vi "WF phase diversity_MATLAB_Correction_loop_AndorSDK.vi"() -> ()   [LabVIEW 2018]
uses:
  <userlib>/WaveKit.lib/Controls/Wavefront Corrector states - ONE.ctl
  <userlib>/WaveKit.lib/Classes/WavefrontCorrector/WavefrontCorrector.lvclass
  <userlib>/WaveKit.lib/Classes/WavefrontCorrectorSet/WavefrontCorrectorSet.lvclass
  <vilib>/Analysis/1siggen.llb/Ramp Pattern by Samples.vi
  <vilib>/Utility/file.llb/Read From Spreadsheet File (DBL).vi
  <vilib>/Analysis/1siggen.llb/Ramp Pattern by Delta.vi
  <vilib>/Analysis/NI_AALBase.lvlib
panel:
  out "Error out tbd":errorcluster
  in  "Tab Control":T1(tab)
  in  "Offset command file":path=path "D:/SystemAlignment/system_aberration_20200627.dat"
  in  "Initial haso file":path=path "D:/SystemAlignment/system_aberration_residual_20200627.has"
  out "# of Phase":i32
  in  "DM configuration file":path=path "C:/Program Files (x86)/Imagine Optic/Configuration Files/WaveFrontCorrector_mirao52-e_0326.dat"
  out "DM Initial State":T2[](array[typedef])
  out "DM ActuatorsNumber":i32
  out "Error out":errorcluster
  in  "Error in":errorcluster
  in  "EMCCD trigger port":tag="Dev1/port0/line0"
  in  "Cooler set to Temperature":i32=-60
  in  "Trigger":u32(ring)=1 items=["Internal", "External"]
  out "Return from CheckTimings":u32
  out "Calculated Exposure Value":sgl format="%.2f"
  out "Return from SetTemperature":u32
  out "Cooling":i32
  out "Return from Initialize":u32
  out "Detector X Pixels":i32
  out "Detector Y Pixels":i32
  in  "Initialize EMCCD?":bool=TRUE
  in  "Turn off cooler when finished?":bool
  in  "Initial Zer coeff":dbl[](array[numeric])=[0.2, 0.2]
  in  "Initial Zer index":dbl[](array[numeric])=[4.0, 5.0]
  out "Initial Zer coeff\nRandomly generated":dbl[](array[numeric])
  out "Initial Zer index (starting from 4)\nrandomly generated":dbl[](array[numeric])
  in  "aberration tolerance":dbl=0.1 format="%#_13g"
  in  "aberration threshold":dbl=0.25 format="%#_13g"
  in  "?":enum16{"input manually ", "randomly generated"}(ring)
  in  "max random order":i64=9
  in  "NOT YET: Data Acquisition Iteration #":i32=1
  in  "Zern index in 2":i32[](array[numeric])=[3, 4, 5, 6, 7, 8]
  in  "Zern coef in 2":sgl[](array[numeric])=[0.2, 0.5, 0.0, 0.0, 0.0, 0.0]
  in  "Zern index in 3":i32[](array[numeric])=[3, 4, 5, 6, 7, 8]
  in  "Zern coef in 3":sgl[](array[numeric])=[0.2, 0.0, 0.0, 0.0, 0.0, 0.0]
  in  "Zern index in 4":i32[](array[numeric])=[3, 4, 5, 6, 7, 8]
  in  "Zern coef in 4":sgl[](array[numeric])=[0.2, 0.0, 0.0, 0.0, 0.0, 0.0]
  in  "Zern index in 5":i32[](array[numeric])=[3, 4, 5, 6, 7, 8]
  in  "Zern coef in 5":sgl[](array[numeric])=[0.0, 0.0, 0.0, 0.0, 0.0, -0.2]
  in  "Andor Picture/notes save to path":path=path "D:/YD/test/test1"
  in  "base name (no \"_\" in the end)":string="beads_test"
  in  "Pics/phase":dbl=2.0
  in  "camera exposure time (s)":string="0.02"
  in  "# of Phase":i32=5
  in  "COMMAND matrix path":path=path "D:/SystemAlignment/CM_20200711_0p5x6.aomc"
  in  "488 shutter":refnum<k7>(container)
  in  "?":bool
  out "phase diversity file name":string
  out "Corrected Picture name":string
  in  "Use GPU":bool=TRUE
  in  "Show Recon":bool=TRUE
  in  "Show Input":bool
  in  "Background Value":u32=310
  in  "Crop Size of image":u32=512
  in  "Gamma Value":dbl=1e-06
  in  "Iteration Number":u32=10
  in  "Zernike Order":u32=21
  in  "Number for average":u32=2
  in  "Number of Phase":u32=2
  in  "Run MATLAB or correction?":bool=TRUE
  in  "Keep Reconstructed Defocus component?":bool
  # "matlab module :\nC:\\Control Software\\LabviewControl\\sub_vis_Wavekit\\recon_zern_fileIO_MATLAB_v2.vi"
  # "Cooler is off for testing"
  # "If Pics/phase is 2:\npicture order:\n\noffset+aberr *2\nphase diversity *8\n\nground truth *1\noffset+aberr *1\ncorrected *2 but the last one cannot be seen in imagej"
  # "Randomly Generate Initial Zernike, enter here:"
  # "Manually input, enter here:"
  # "Andor Camera Settings"
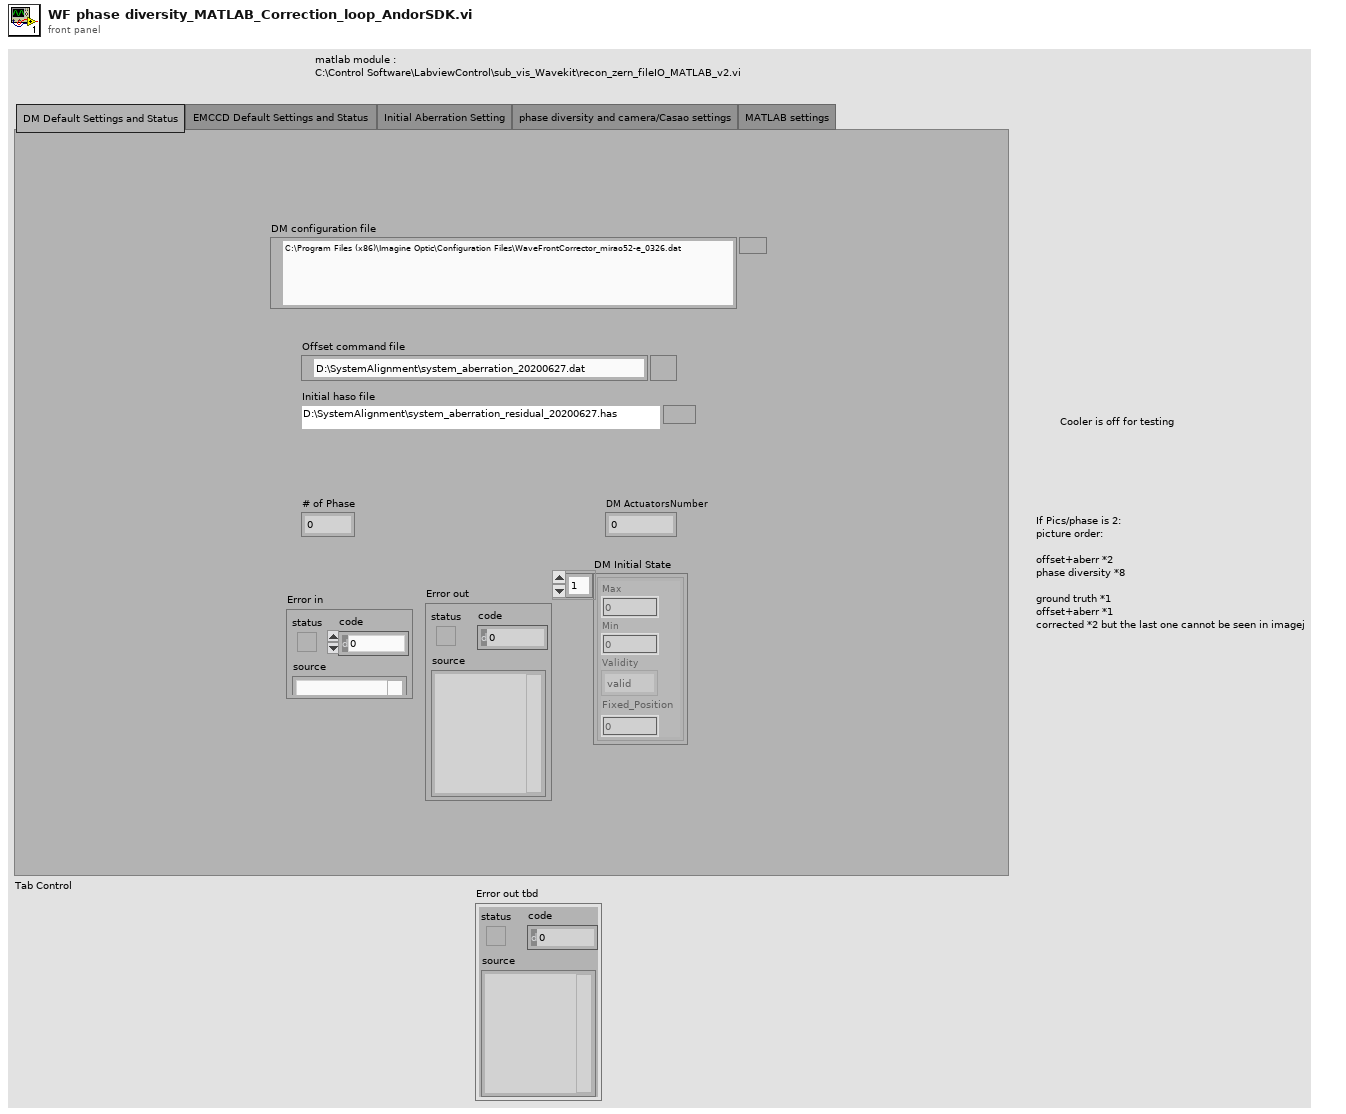
[diagram p1: front panel]
types:
  T1 = enum32{"DM Default Settings and Status", "EMCCD Default Settings and Status ", "Initial Aberration Setting", "phase diversity and camera/Casao settings", "MATLAB settings"}
  T2 = typedef "Wavefront Corrector states - ONE.ctl" = cluster{"Max":sgl, "Min":sgl, "Validity":enum16{"valid", "fixed", "invalid"}, "Fixed_Position":sgl}
  T3 = typedef "Error Code Enum typedef.ctl" = enum32{"N/A (0)", "DRV_ERROR_CODES", "DRV_SUCCESS", "DRV_VXDNOTINSTALLED", "DRV_ERROR_SCAN", "DRV_ERROR_CHECK_SUM", "DRV_ERROR_FILELOAD", "DRV_UNKNOWN_FUNC", "DRV_ERROR_VXD_INIT", "DRV_ERROR_ADDRESS", "DRV_ERROR_PAGELOCK", "DRV_ERROR_PAGEUNLOCK", "DRV_ERROR_BOARDTEST", "DRV_ERROR_ACK", "DRV_ERROR_UP_FIFO", "DRV_ERROR_PATTERN", "N/A (16)", "DRV_ACQUISITION_ERRORS", "DRV_ACQ_BUFFER", "DRV_ACQ_DOWNFIFO_FULL", "DRV_PROC_UNKONWN_INSTRUCTION", "DRV_ILLEGAL_OP_CODE", "DRV_KINETIC_TIME_NOT_MET", "DRV_ACCUM_TIME_NOT_MET", "DRV_NO_NEW_DATA", "N/A (25)", "DRV_SPOOLERROR", "N/A (27)", "N/A (28)", "N/A (29)", "N/A (30)", "N/A (31)", "N/A (32)", "DRV_TEMPERATURE_CODES", "DRV_TEMPERATURE_OFF", "DRV_TEMPERATURE_NOT_STABILIZED", "DRV_TEMPERATURE_STABILIZED", "DRV_TEMPERATURE_NOT_REACHED", "DRV_TEMPERATURE_OUT_RANGE", "DRV_TEMPERATURE_NOT_SUPPORTED", "DRV_TEMPERATURE_DRIFT", "N/A (41)", "N/A (42)", "N/A (43)", "N/A (44)", "N/A (45)", "N/A (46)", "N/A (47)", "N/A (48)", "DRV_GENERAL_ERRORS", "DRV_INVALID_AUX", "DRV_COF_NOTLOADED", "DRV_FPGAPROG", "DRV_FLEXERROR", "DRV_GPIBERROR", "N/A (55)", "N/A (56)", "N/A (57)", "N/A (58)", "N/A (59)", "N/A (60)", "N/A (61)", "N/A (62)", "N/A (63)", "DRV_DATATYPE", "DRV_DRIVER_ERRORS", "DRV_P1INVALID", "DRV_P2INVALID", "DRV_P3INVALID", "DRV_P4INVALID", "DRV_INIERROR", "DRV_COFERROR", "DRV_ACQUIRING", "DRV_IDLE", "DRV_TEMPCYCLE", "DRV_NOT_INITIALIZED", "DRV_P5INVALID", "DRV_P6INVALID", "DRV_INVALID_MODE", "DRV_INVALID_FILTER", "DRV_I2CERRORS", "DRV_I2CDEVNOTFOUND", "DRV_I2CTIMEOUT", "DRV_P7INVALID", "N/A (84)", "N/A (85)", "N/A (86)", "N/A (87)", "N/A (88)", "N/A (89)", "DRV_IOCERROR", "DRV_VRMVERSIONERROR"}
  T4 = typedef "NI_Matrix.lvlib/RealMatrix.ctl" = dbl[][]
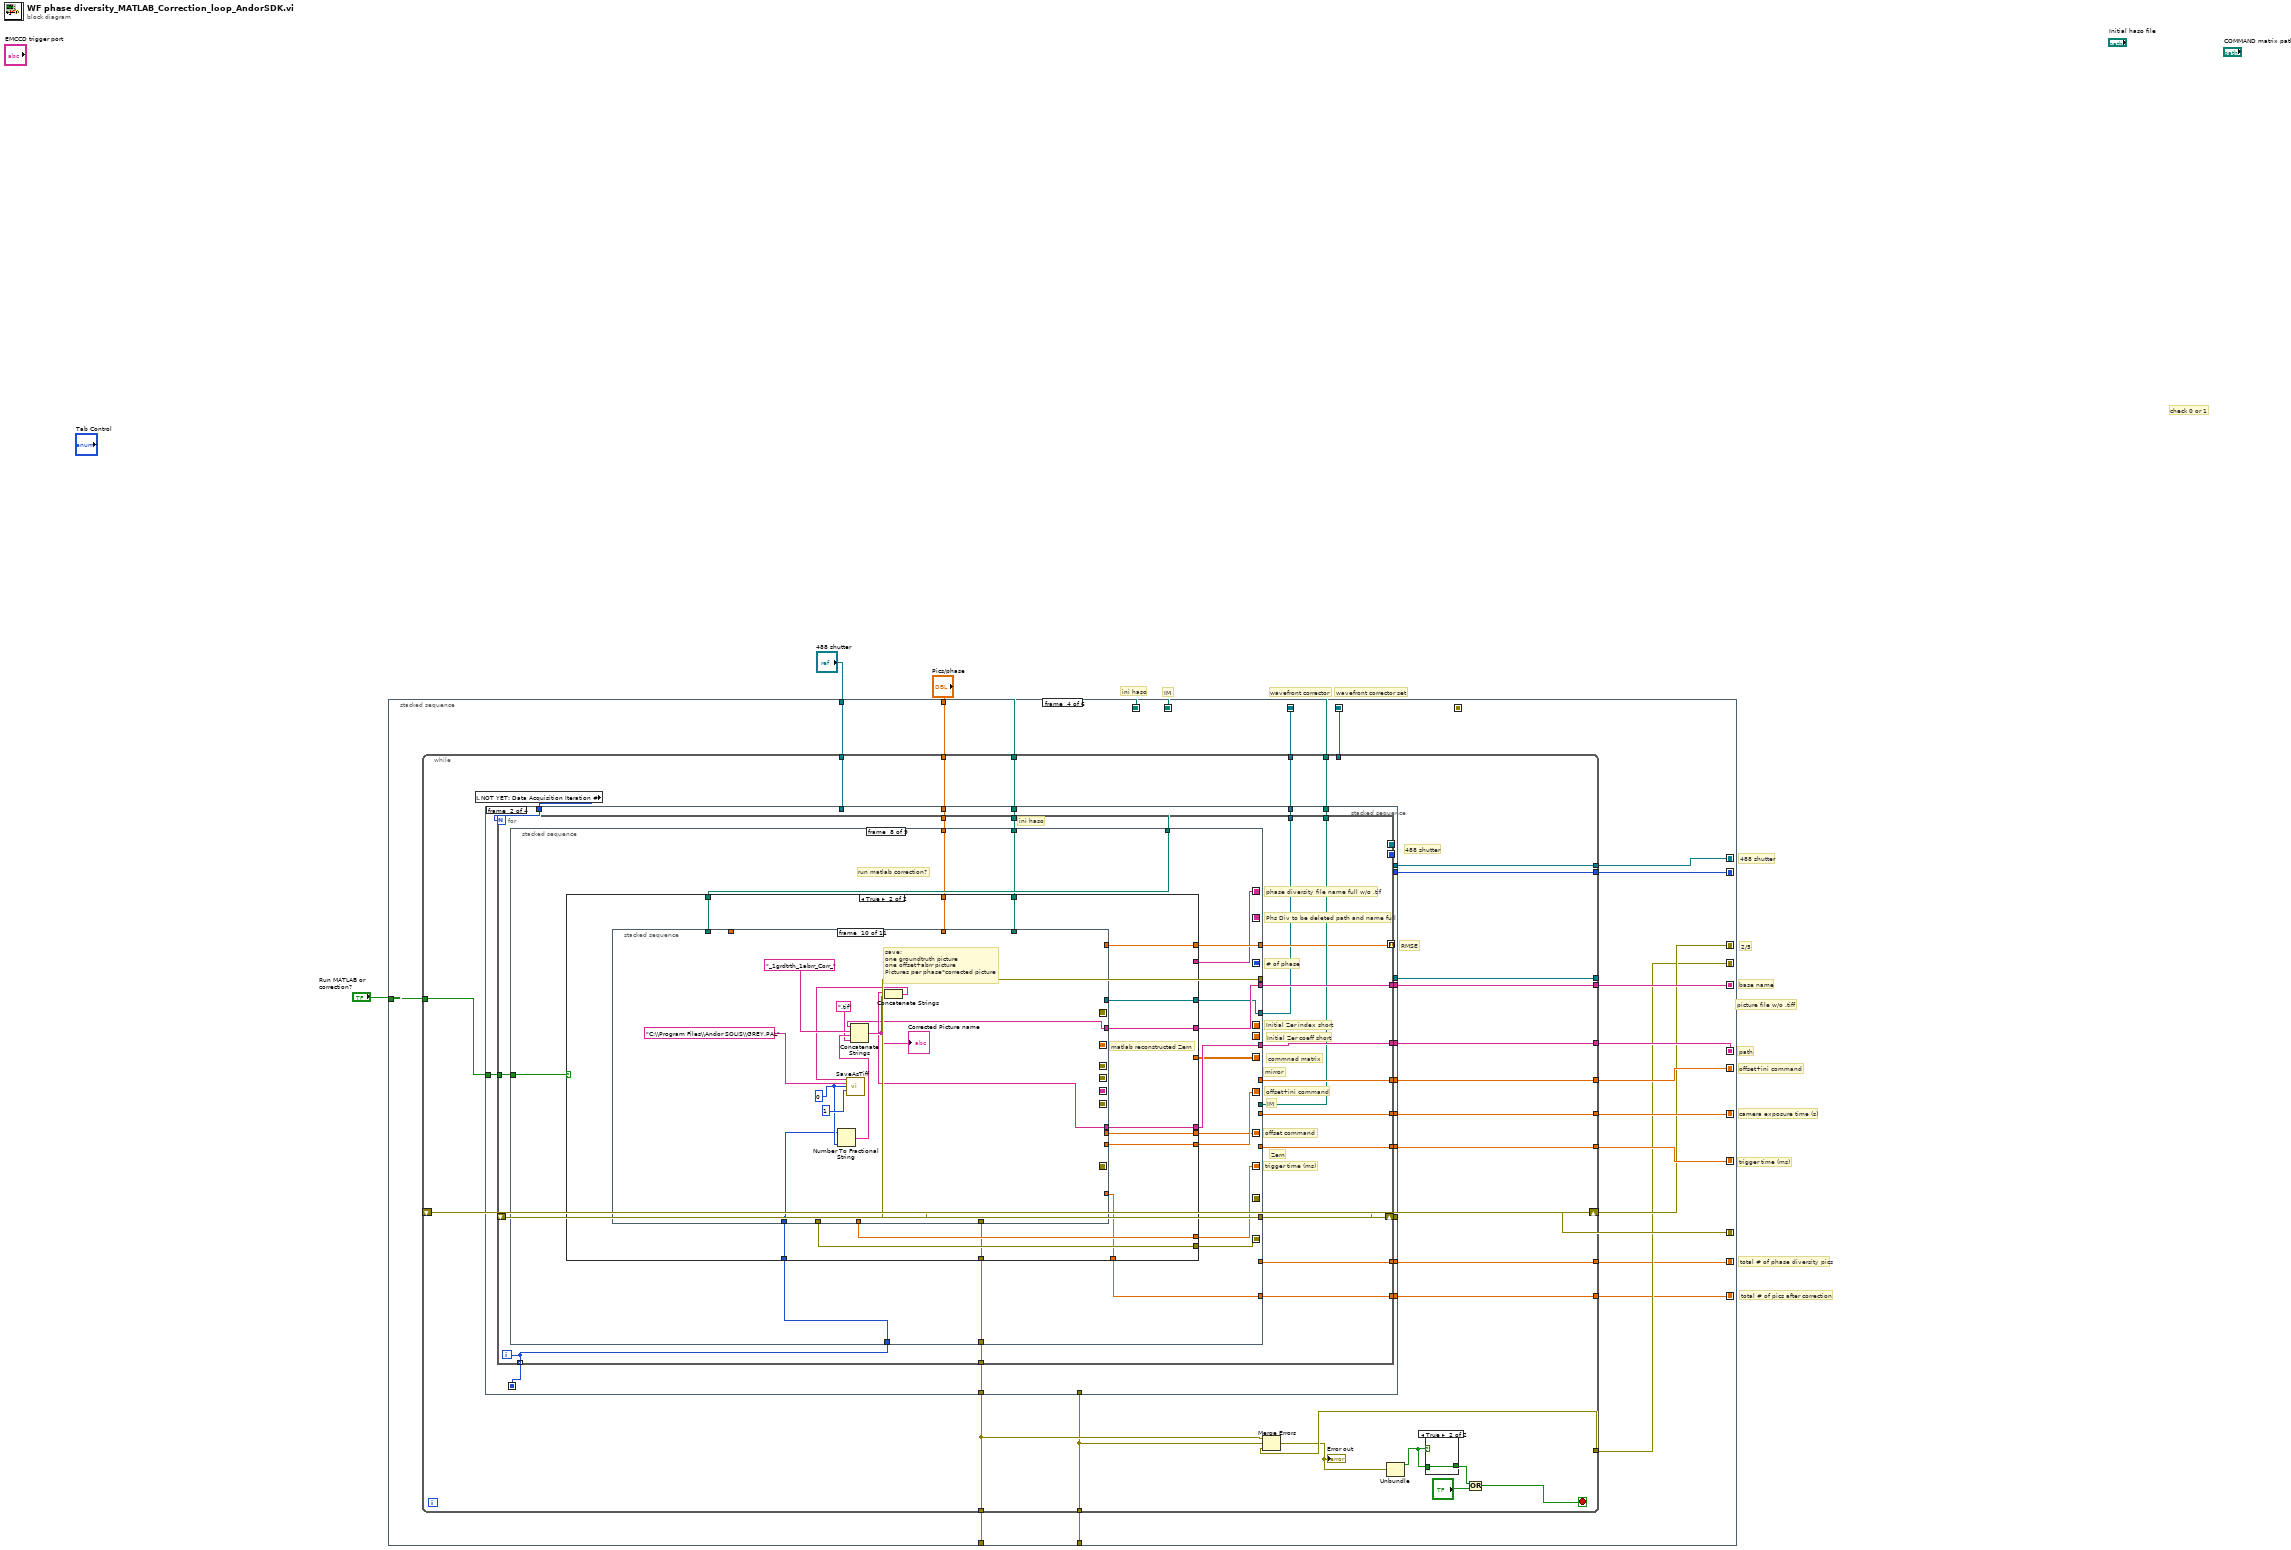
[diagram p0: block diagram]
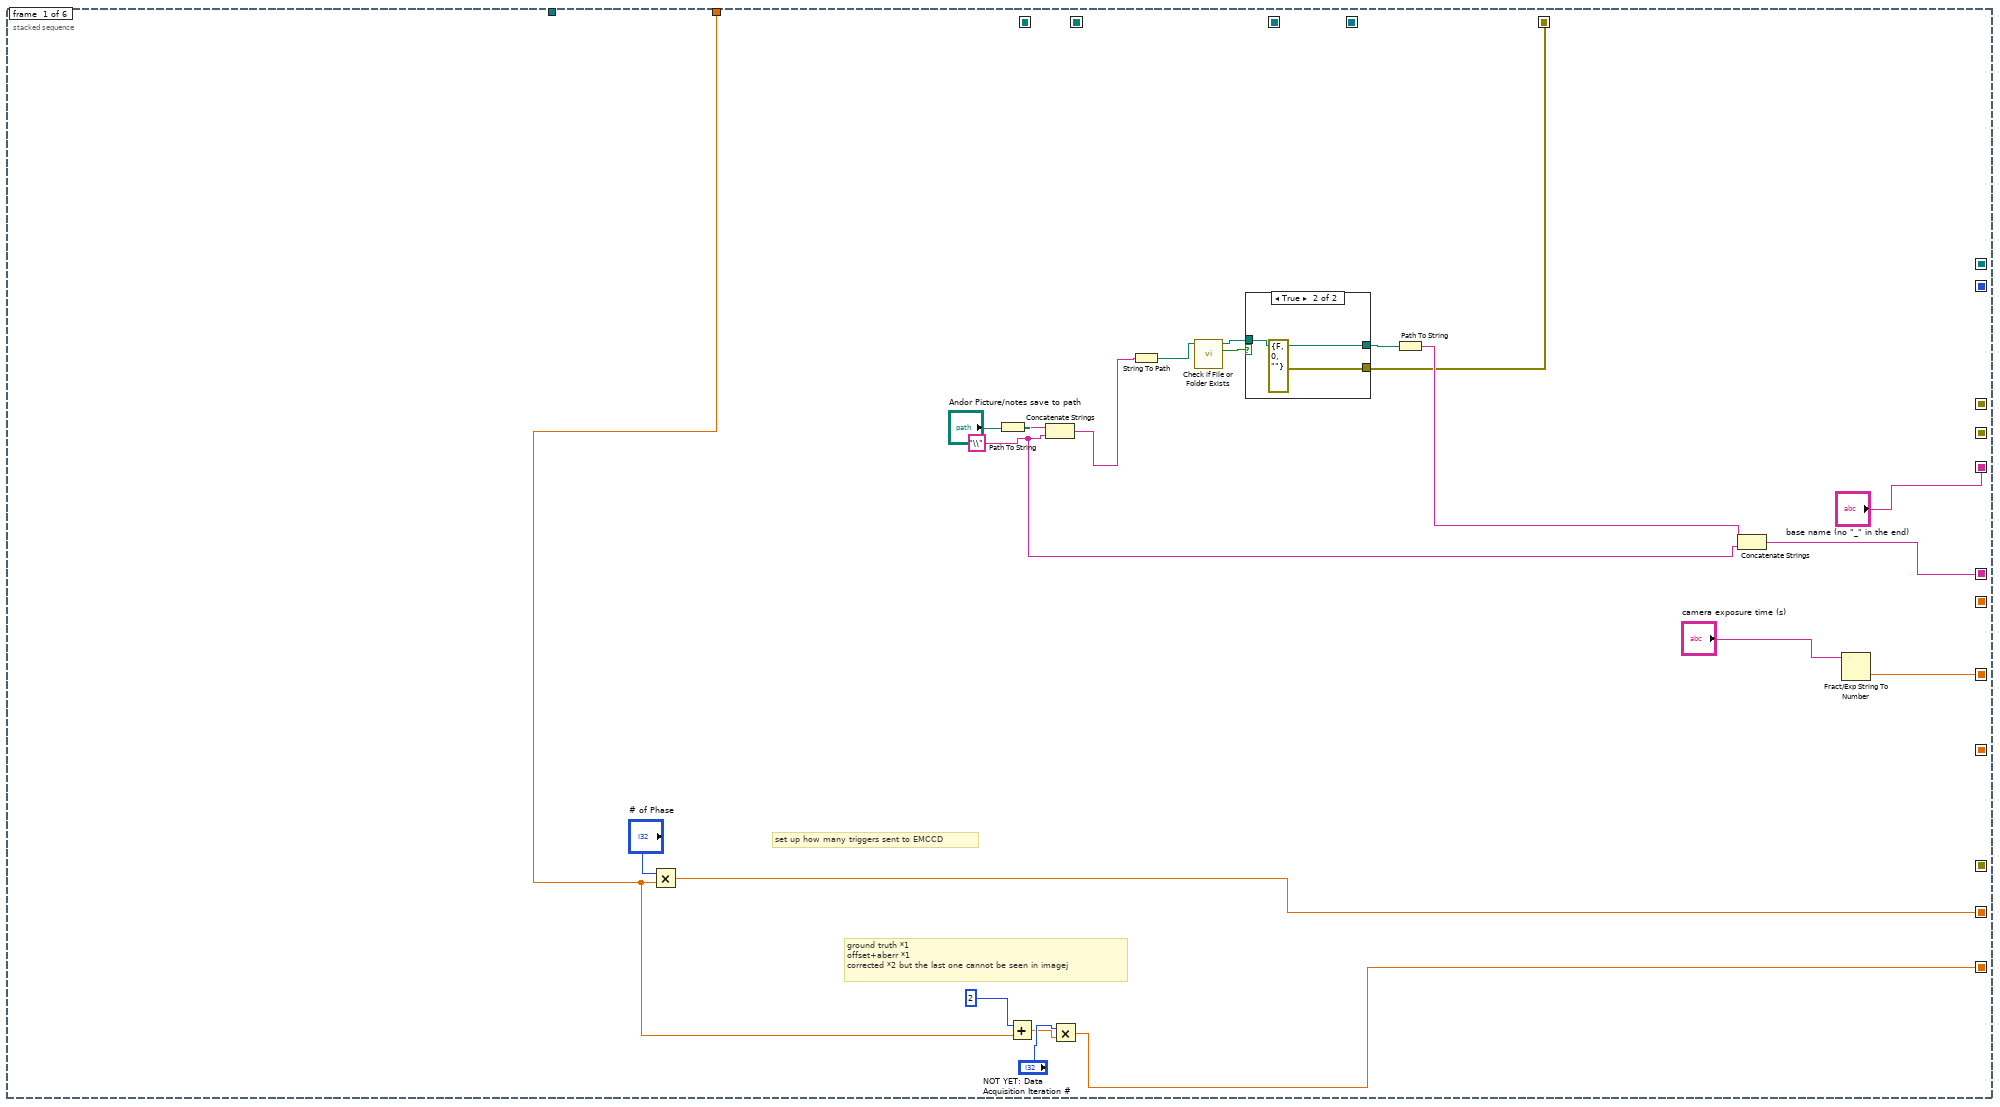
[diagram p2: hidden frame]
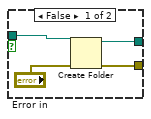
[diagram p3: hidden frame]
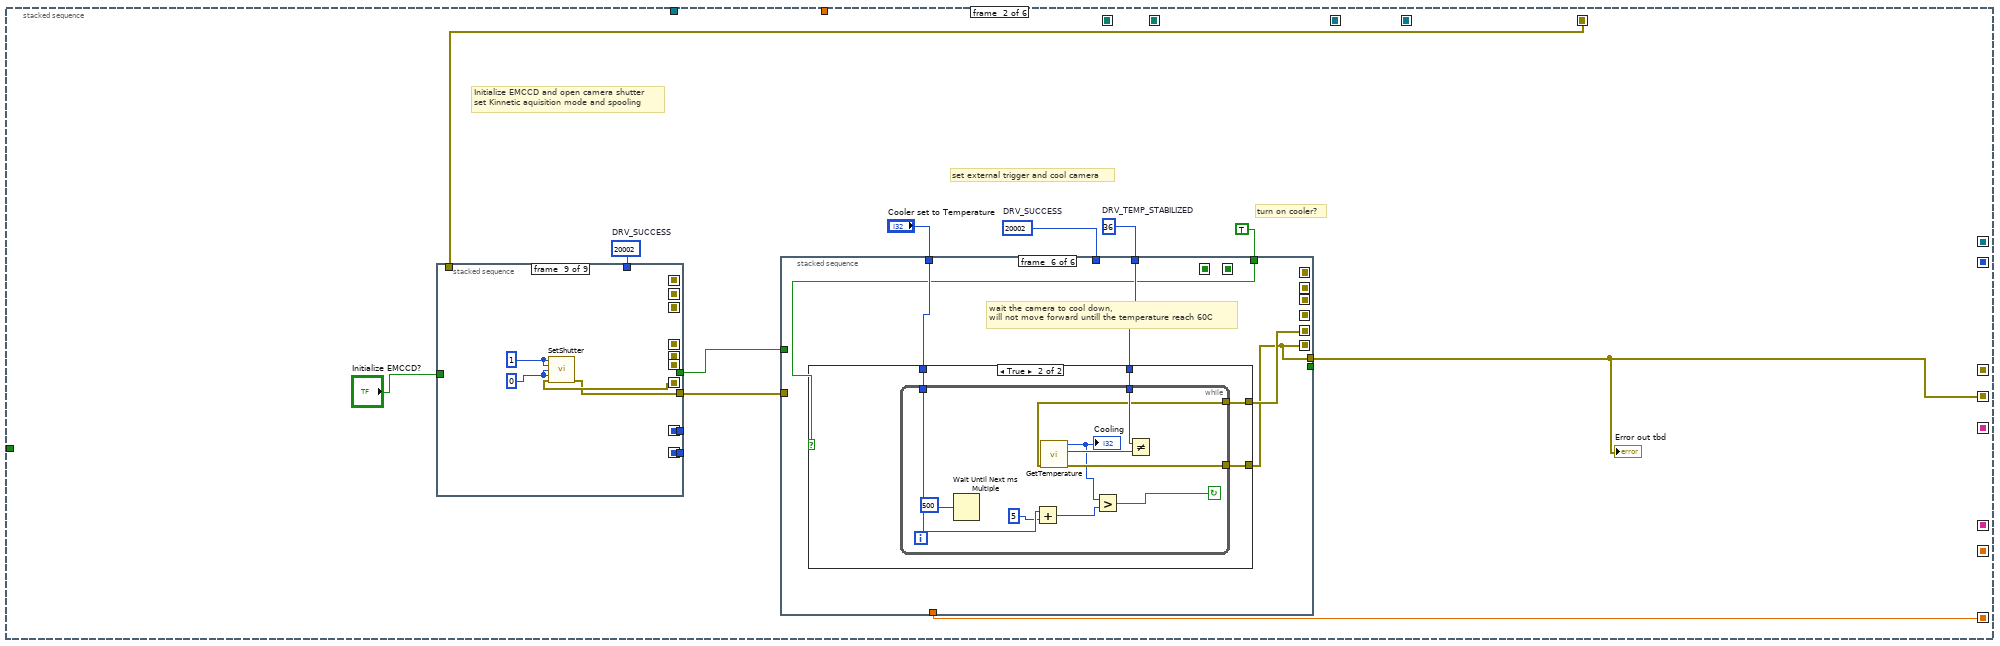
[diagram p4: hidden frame]
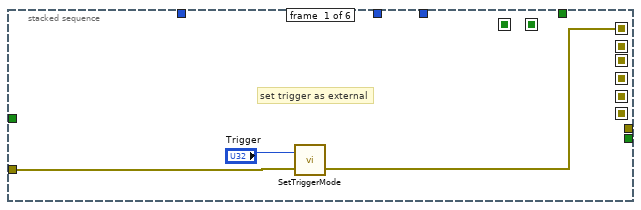
[diagram p5: hidden frame]
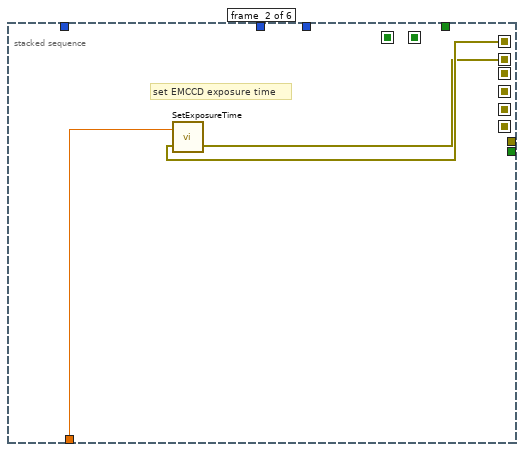
[diagram p6: hidden frame]
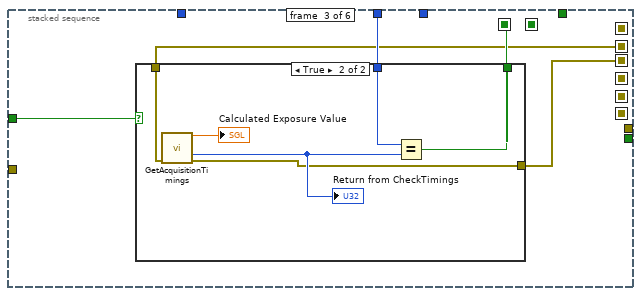
[diagram p7: hidden frame]
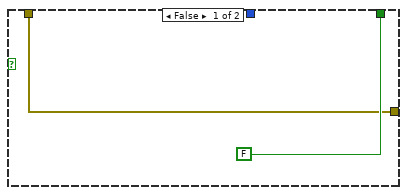
[diagram p8: hidden frame]
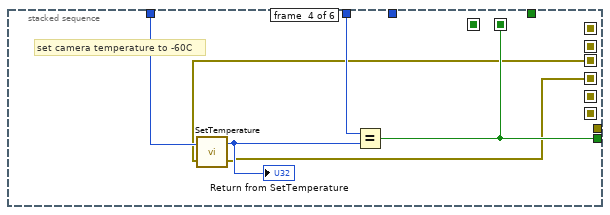
[diagram p9: hidden frame]
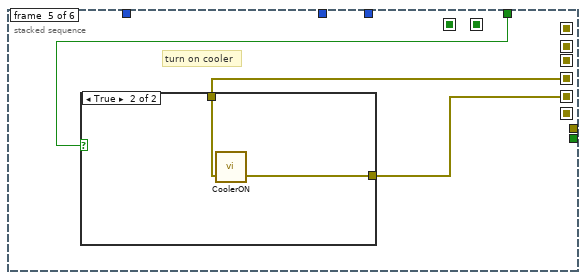
[diagram p10: hidden frame]
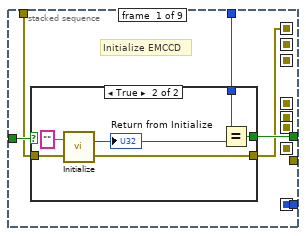
[diagram p13: hidden frame]
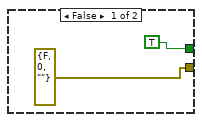
[diagram p14: hidden frame]
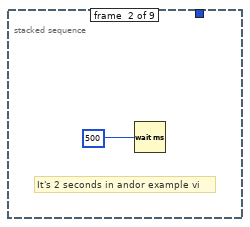
[diagram p15: hidden frame]
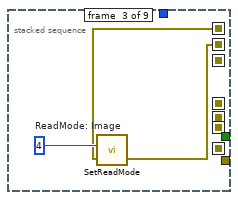
[diagram p16: hidden frame]
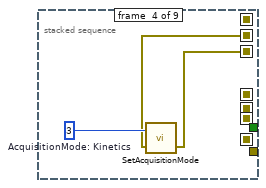
[diagram p17: hidden frame]
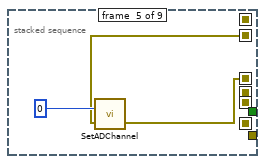
[diagram p18: hidden frame]
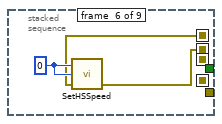
[diagram p19: hidden frame]
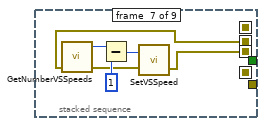
[diagram p20: hidden frame]
diagram:
  # "2/5"
  # "total # of phase diversity pics"
  # "picture file w/o .tiff"
  # "total # of pics after correction"
  # "wavefront corrector set"
  # "wavefront corrector"
  # "488 shutter"
  # "trigger time (ms)"
  # "offset+ini command"
  # "camera exposure time (s)"
  # "IM"
  # "ini haso"
  # "path"
  # "base name"
  # "check 0 or 1"
  n1 = stacked-sequence {
    seq-local: [w5 _ _ _ _ _] -> [_ _ _ w174 _ _]
    seq-local: ["base name (no \"_\" in the end)" _ _ _ _ _] -> [_ _ _ w173 _ _]
    seq-local: [_ _ w154 _ _ _] -> [_ _ _ w172 _ _]
    seq-local: [_ _ w153 _ _ _] -> [_ _ _ w167 _ _]
    seq-local: [w19 _ _ _ _ _] -> [_ w35 _ w171 _ _]
    seq-local: [_ _ w139 _ _ _] -> [_ _ _ w159 _ _]
    seq-local: [_ _ _ w170 _ _] -> [_ _ _ _ _ _]
    seq-local: [_ _ _ w169 _ _] -> [_ _ _ _ _ _]
    seq-local: [_ _ _ w168 _ _] -> [_ _ _ _ _ w643]
    seq-local: [_ _ _ w162 _ _] -> [_ _ _ _ _ _]
    seq-local: [_ _ _ w165 _ _] -> [_ _ _ _ _ _]
    seq-local: [_ _ w138 _ _ _] -> [_ _ _ w160 _ w645]
    seq-local: [_ _ w137 _ _ _] -> [_ _ _ w158 _ w644]
    seq-local: [w16 _ _ _ _ _] -> [_ _ _ w155 _ _]
    seq-local: [_ w31 _ _ _ _] -> [_ _ w136 w157 _ _]
    seq-local: [w15 _ _ _ _ _] -> [_ _ _ w156 _ _]
    seq-local: [w4 _ _ _ _ _] -> [_ w32 _ _ _ _]
    tunnel: "Pics/phase" -> [w13 _ _ w175 _ _]
    tunnel: "Run MATLAB or correction?" -> [_ _ _ w166 _ _]
    tunnel: [_ _ _ w164 _ _] -> _
    tunnel: [_ _ _ w163 _ _] -> _
    tunnel: "488 shutter" -> [_ _ _ w161 _ w646]
    frame #0 {
      w6 = "\\"
      # "set up how many triggers sent to EMCCD"
      # "ground truth *1\noffset+aberr *1\ncorrected *2 but the last one cannot be seen in imagej"
      n2 = Multiply(x="# of Phase", y=w13) -> (x*y=w15:dbl)
      n3 = Path To String(path="Andor Picture/notes save to path") -> (string=w21:string)
      n4 = Add(x=2, y=w13) -> (x+y=w17:dbl)
      n5 = Concatenate Strings(w21, w6) -> (w8:string)
      n6 = Multiply(x="NOT YET: Data Acquisition Iteration #", y=w17) -> (x*y=w16:dbl)
      n7 = String To Path(string=w8) -> (path=w12:path)
      n8 = call <vilib>:"Check if File or Folder Exists.vi"("path"=w12) -> ("file or folder exists?"=w10:bool, "dup path"=w11:path)  [unwired: 8 in, 1 out]
      n9 = case shown="True" w10 {
        tunnel: w11 -> [w28 w30]
        tunnel: [w27 w30] -> w9
        tunnel: [w25 errorcluster {"status"=FALSE, "code"=0, "source"=""} ("Error in 3")] -> w4
        frame False {
          n10 = Create Folder(path (use dialog)=w28, error in="Error in") -> (created path=w27:path, error out=w25:errorcluster)  [unwired: 1 in, 1 out]
        }
        frame True {
        }
      }
      n11 = Path To String(path=w9) -> (string=w7:string)
      n12 = Concatenate Strings(w7, w6) -> (w5:string)
      n13 = Fract/Exp String To Number(string="camera exposure time (s)") -> (number=w19:dbl)  [unwired: 3 in, 1 out]
    }
    frame #1 {
      w37 = 36  # DRV_TEMP_STABILIZED
      w39 = 20002  # DRV_SUCCESS
      w41 = 20002  # DRV_SUCCESS
      # "turn on cooler?"
      # "set external trigger and cool camera"
      # "Initialize EMCCD and open camera shutter\nset Kinnetic aquisition mode and spooling"
      n14 = stacked-sequence {
        seq-local: [_ _ _ _ _ _ _ w125 _] -> [_ _ _ _ _ _ _ _ _]
        seq-local: [_ _ _ _ _ _ _ w127 _] -> [_ _ _ _ _ _ _ _ _]
        seq-local: [w95 _ _ _ _ _ _ _ _] -> [_ _ w108 _ _ _ _ _ _]
        seq-local: [_ _ w107 _ _ _ _ _ _] -> [_ _ _ w111 _ _ _ _ _]
        seq-local: [_ _ _ w110 _ _ _ _ _] -> [_ _ _ _ w113 _ _ _ _]
        seq-local: [_ _ _ _ w114 _ _ _ _] -> [_ _ _ _ _ w117 _ _ _]
        seq-local: [_ _ _ _ _ w116 _ _ _] -> [_ _ _ _ _ _ w121 _ _]
        seq-local: [_ _ _ _ _ _ w119 _ _] -> [_ _ _ _ _ _ _ w130 _]
        seq-local: [_ _ _ _ _ _ _ w128 _] -> [_ _ _ _ _ _ _ _ w133]
        tunnel: w41 -> [w97 _ _ _ _ _ _ _ _]
        tunnel: [w96 _ _ _ _ _ _ _ _] -> w40
        tunnel: [_ _ _ _ _ _ _ w125 _] -> _
        tunnel: [_ _ _ _ _ _ _ w127 _] -> _
        tunnel: [_ _ _ _ _ _ _ _ w132] -> w36
        tunnel: "Initialize EMCCD?" -> [w94 _ _ _ _ _ _ _ _]
        tunnel: w32 -> [w93 _ _ _ _ _ _ _ _]
        frame #0 {
          # "Initialize EMCCD"
          n15 = case shown="True" w94 {
            tunnel: w97 -> [_ w103]
            tunnel: [TRUE w102] -> w96
            tunnel: [errorcluster {"status"=FALSE, "code"=0, "source"=""} ("Error in 2") w101] -> w95
            tunnel: w93 -> [_ w100]
            frame False {
            }
            frame True {
              n16 = call <userlib>:"Initialize.vi"("error in (no error)"=w100, "directory (\"\")"="" ("directory (\"\")")) -> ("error out"=w101:errorcluster, "DLL error code"=w105:u32)
              "Return from Initialize" <- w105
              n17 = Equal?(x=w103, y=w105) -> (x = y?=w102:bool)
            }
          }
        }
        frame #1 {
          # "It's 2 seconds in andor example vi"
          n18 = Wait (ms)(milliseconds to wait=u32 500) -> ()  [unwired: 1 out]
        }
        frame #2 {
          w109 = u16 4  # ReadMode: Image
          n19 = call <userlib>:"SetReadMode.vi"("error in (no error)"=w108, "mode"=w109) -> ("error out"=w107:errorcluster)  [unwired: 1 out]
        }
        frame #3 {
          w112 = u16 3  # AcquisitionMode: Kinetics
          n20 = call <userlib>:"SetAcquisitionMode.vi"("error in (no error)"=w111, "mode"=w112) -> ("error out"=w110:errorcluster)  [unwired: 1 out]
        }
        frame #4 {
          n21 = call <userlib>:"SetADChannel.vi"("error in (no error)"=w113, "channel"=0) -> ("error out"=w114:errorcluster)  [unwired: 1 out]
        }
        frame #5 {
          w118 = 0
          n22 = call <userlib>:"SetHSSpeed.vi"("error in (no error)"=w117, "index"=w118, "type"=w118) -> ("error out"=w116:errorcluster)  [unwired: 1 in, 1 out]
        }
        frame #6 {
          n23 = call <userlib>:"GetNumberVSSpeeds.vi"("error in (no error)"=w121) -> ("error out"=w120:errorcluster, "number"=w124:i32)  [unwired: 2 in, 1 out]
          n24 = Subtract(x=w124, y=1) -> (x-y=w122:i32)
          n25 = call <userlib>:"SetVSSpeed.vi"("error in (no error)"=w120, "index"=w122) -> ("error out"=w119:errorcluster)  [unwired: 1 out]
        }
        frame #7 {
          w125 = 1002
          w131 = 1
          n26 = call <userlib>:"GetDetector.vi"("error in (no error)"=w130) -> ("error out"=w129:errorcluster, "ypixels"=→"Detector Y Pixels":i32, "xpixels"=w127:i32)  [unwired: 3 in, 1 out]
          "Detector X Pixels" <- w127
          n27 = call <userlib>:"SetImage.vi"("hbin"=w131, "vbin"=w131, "hstart"=w131, "hend"=w125, "vstart"=w131, "vend"=w125, "error in (no error)"=w129) -> ("error out"=w128:errorcluster)  [unwired: 19 in, 1 out]
        }
        frame #8 {
          w134 = 0
          w135 = 1
          n28 = call <userlib>:"SetShutter.vi"("type"=w135, "mode"=w135, "closingtime"=w134, "openingtime"=w134, "error in (no error)"=w133) -> ("error out"=w132:errorcluster)  [unwired: 9 in, 1 out]
        }
      }
      n29 = stacked-sequence {
        seq-local: [_ _ w50 _ _ _] -> [_ _ _ _ _ _]
        seq-local: [_ _ _ w63 _ _] -> [_ _ _ _ _ _]
        seq-local: [w42 _ _ _ _ _] -> [_ w47 _ _ _ _]
        seq-local: [_ w46 _ _ _ _] -> [_ _ w49 _ _ _]
        seq-local: [_ _ w48 _ _ _] -> [_ _ _ w62 _ _]
        seq-local: [_ _ _ w61 _ _] -> [_ _ _ _ w69 _]
        seq-local: [_ _ _ _ w68 _] -> [_ _ _ _ _ w75]
        seq-local: [_ _ _ _ _ w73] -> [_ _ _ _ _ _]
        tunnel: w39 -> [_ _ w52 w66 _ _]
        tunnel: "Cooler set to Temperature" -> [_ _ _ w64 _ w76]
        tunnel: w37 -> [_ _ _ _ _ w77]
        tunnel: [_ _ _ w63 _ _] -> _
        tunnel: w40 -> [_ _ w51 _ _ _]
        tunnel: w36 -> [w43 _ _ _ _ _]
        tunnel: [_ _ _ _ _ w73] -> w31
        tunnel: w35 -> [_ w45 _ _ _ _]
        tunnel: TRUE -> [_ _ _ _ w67 w74]
        frame #0 {
          # "set trigger as external"
          n30 = call <userlib>:"SetTriggerMode.vi"("error in (no error)"=w43, "mode"="Trigger") -> ("error out"=w42:errorcluster)  [unwired: 1 out]
        }
        frame #1 {
          # "set EMCCD exposure time"
          n31 = call <userlib>:"SetExposureTime.vi"("error in (no error)"=w47, "time"=w45) -> ("error out"=w46:errorcluster)  [unwired: 1 out]
        }
        frame #2 {
          n32 = case shown="True" w51 {
            tunnel: w52 -> [_ w58]
            tunnel: [FALSE w60] -> w50
            tunnel: w49 -> [w53 w56]
            tunnel: [w53 w55] -> w48
            frame False {
            }
            frame True {
              n33 = call <userlib>:"GetAcquisitionTimings.vi"("error in (no error)"=w56) -> ("exposure"=→"Calculated Exposure Value":sgl, "DLL error code"=w57:u32, "error out"=w55:errorcluster)  [unwired: 10 in, 2 out]
              "Return from CheckTimings" <- w57
              n34 = Equal?(x=w58, y=w57) -> (x = y?=w60:bool)
            }
          }
        }
        frame #3 {
          # "set camera temperature to -60C"
          n35 = call <userlib>:"SetTemperature.vi"("error in (no error)"=w62, "temperature"=w64) -> ("error out"=w61:errorcluster, "DLL error code"=w65:u32)
          "Return from SetTemperature" <- w65
          n36 = Equal?(x=w66, y=w65) -> (x = y?=w63:bool)
        }
        frame #4 {
          # "turn on cooler"
          n37 = case shown="True" w67 {
            tunnel: w69 -> [w70 w72]
            tunnel: [w70 w71] -> w68
            frame False {
            }
            frame True {
              n38 = call <userlib>:"CoolerON.vi"("error in (no error)"=w72) -> ("error out"=w71:errorcluster)  [unwired: 1 in, 1 out]
            }
          }
        }
        frame #5 {
          # "wait the camera to cool down,\nwill not move forward untill the temperature reach 60C"
          n39 = case shown="True" w74 {
            tunnel: w77 -> [_ w82]
            tunnel: w76 -> [_ w81]
            tunnel: w75 -> [w78 w80]
            tunnel: [w78 w79] -> w73
            frame False {
            }
            frame True {
              n40 = while {
                tunnel: w82 -> [w91]
                tunnel: w81 -> [w86]
                tunnel: w80 -> [w89]
                tunnel: [w88] -> w79
                stop <- w83 continue-if-true
                n41 = Wait Until Next ms Multiple(millisecond multiple=u32 500) -> ()  [unwired: 1 out]
                n42 = Add(x=w86, y=5) -> (x+y=w84:i32)
                n43 = call <userlib>:"GetTemperature.vi"("error in (no error)"=w89) -> ("error out"=w88:errorcluster, "status"=w90:T3, "temperature"=w87:i32)  [unwired: 3 in, 1 out]
                "Cooling" <- w87
                n44 = Greater?(x=w87, y=w84) -> (0:w83:bool)
                n45 = Not Equal?(x=w91, y=w90) -> ()  [unwired: 1 out]
              }
            }
          }
        }
      }
      "Error out tbd" <- w31
    }
    frame #2 {
      # "Initialize CASAO"
      n46 = call <userlib>:"LVClass_WavefrontCorrectorSet ctor.vi"("WavefrontCorrectorSet in"=refnum<class "WavefrontCorrectorSet.lvclass"> refnum, "PathToWavefrontCorrectorSetupFile"="DM configuration file", "error in (no error)"=w136) -> ("WavefrontCorrectorSet out"=w143:refnum<class "WavefrontCorrectorSet.lvclass">, "error out"=w152:errorcluster)  [unwired: 11 in]
      n47 = call <userlib>:"LVClass_WavefrontCorrector ctor.vi"("WavefrontCorrector in"=refnum<class "WavefrontCorrector.lvclass"> refnum, "PathToWavefrontCorrectorSetupFile"="DM configuration file", "error in (no error)"=w152) -> ("WavefrontCorrector out"=w147:refnum<class "WavefrontCorrector.lvclass">, "error out"=w146:errorcluster)  [unwired: 11 in]
      n48 = call <userlib>:"LVClass_WavefrontCorrector Init.vi"("WavefrontCorrector in"=w147, "set_init_state_from_config_file"=TRUE, "error in (no error)"=w146) -> ("WavefrontCorrector out"=w141:refnum<class "WavefrontCorrector.lvclass">, "error out"=w145:errorcluster)  [unwired: 11 in]
      n49 = call <userlib>:"LVClass_WavefrontCorrectorSet get nb of actuators.vi"("WavefrontCorrectorSet in"=w143, "error in (no error)"=w145) -> ("WavefrontCorrectorSet out"=w137:refnum<class "WavefrontCorrectorSet.lvclass">, "ActuatorsNumber"=→"DM ActuatorsNumber":i32, "error out"=w142:errorcluster)  [unwired: 11 in]
      n50 = call <userlib>:"LVClass_WavefrontCorrector Get Current Preferences.vi"("WavefrontCorrector in"=w141, "error in (no error)"=w142) -> ("WavefrontCorrector out"=w138:refnum<class "WavefrontCorrector.lvclass">, "Mirror preferences.Wavefront Corrector State"=→"DM Initial State":T2[], "error out"=w139:errorcluster)  [unwired: 10 in, 1 out]
      n51 = local read "COMMAND matrix path"() -> (w153:path)
      n52 = local read "Initial haso file"() -> (w154:path)
    }
    frame #3 {
      n53 = while {
        tunnel: w175 -> [w202]
        tunnel: w174 -> [w201]
        tunnel: w173 -> [w200]
        tunnel: w172 -> [w199]
        tunnel: w171 -> [w198]
        tunnel: [w196] -> w170
        tunnel: [w195] -> w169
        tunnel: w167 -> [w193]
        tunnel: w166 -> [w192]
        tunnel: [w191] -> w165
        tunnel: [w190] -> _
        tunnel: [w188] -> w164
        tunnel: [w189] -> w163
        shift-right: [w194] -> w168
        shift-left: w159 -> [w197]
        tunnel: [w187] -> w162
        tunnel: w161 -> [w186]
        tunnel: w160 -> [w185]
        tunnel: w158 -> [_]
        tunnel: w157 -> [w183]
        tunnel: w156 -> [w177]
        tunnel: w155 -> [w176]
        stop <- w179 stop-if-true
        # "488 shutter"
        # "RMSE"
        n54 = local read "NOT YET: Data Acquisition Iteration #"() -> (w184:i32)
        n55 = stacked-sequence {
          seq-local: [_ w218 _ _] -> [_ _ _ w636]
          seq-local: [_ w217 _ _] -> [_ _ _ _]
          seq-local: [w207 _ _ _] -> [_ _ w632 _]
          seq-local: [w208 _ _ _] -> [_ _ w631 _]
          tunnel: w202 -> [_ w230 _ _]
          tunnel: w201 -> [_ w229 _ w635]
          tunnel: w200 -> [_ w228 _ w634]
          tunnel: w199 -> [_ w227 _ _]
          tunnel: w198 -> [_ w226 _ _]
          tunnel: w197 -> [_ w225 _ _]
          tunnel: [_ w224 _ _] -> w196
          tunnel: [_ w223 _ _] -> w195
          tunnel: [_ w222 _ _] -> w194
          tunnel: w193 -> [_ w221 _ _]
          tunnel: w192 -> [_ w220 _ _]
          tunnel: w184 -> [_ w219 _ _]
          tunnel: [_ _ w630 _] -> w190
          tunnel: [_ _ w629 _] -> w191
          tunnel: [_ _ _ w633] -> w188
          tunnel: [_ w216 _ _] -> w189
          tunnel: [w207 _ _ _] -> w187
          tunnel: w186 -> [w206 _ _ _]
          tunnel: w185 -> [_ w215 _ _]
          tunnel: w177 -> [_ w214 _ _]
          tunnel: w176 -> [_ w213 _ _]
          frame #0 {
            # "open the shutter of 488nm laser"
            n56 = property class="MG17Motor"(reference=w206, "HWSerialNum"=85819115.0) -> (reference out=w212:refnum<k7>)  [unwired: 1 in, 1 out]
            n57 = invoke class="MG17Motor" method="StartCtrl"(reference=w212) -> (reference out=w210:refnum<k7>)  [unwired: 2 in, 2 out]
            n58 = invoke class="MG17Motor" method="SC_Enable"(reference=w210, "lChanID"=0) -> (reference out=w207:refnum<k7>, "lChanID"=w208:i32)  [unwired: 2 in, 2 out]
          }
          frame #1 {
            n59 = for {
              N: w219 -> [_]
              tunnel: w230 -> [w247]
              tunnel: w229 -> [w246]
              tunnel: w228 -> [w245]
              tunnel: w227 -> [w244]
              tunnel: w226 -> [w243]
              tunnel: [w241] -> w224
              tunnel: [w240] -> w223
              tunnel: w221 -> [w238]
              tunnel: w220 -> [w237]
              shift-right: [w239] -> w222
              shift-left: w225 -> [w242]
              tunnel: [w236] -> w218 mode=indexing
              tunnel: [w235] -> w217 mode=indexing
              tunnel: [w234] -> w216
              tunnel: w215 -> [w233]
              tunnel: w214 -> [w232]
              tunnel: w213 -> [w231]
              i -> [w235]
              # "Phs Div to be deleted path and name full"
              # "phase diversity file name full w/o .tif"
              # "# of phase"
              # "trigger time (ms)"
              # "offset+ini command"
              # "Initial Zer coeff short"
              # "Initial Zer index short"
              # "mirror"
              # "Zern"
              # "commnad matrix"
              # "ini haso"
              # "IM"
              # "offset command"
              n60 = stacked-sequence {
                seq-local: [_ w259 _ _ _ _ _ _ _] -> [_ _ w279 _ w407 _ _ w470 _]
                seq-local: [_ _ w277 _ _ _ _ _ _] -> [_ _ _ _ w406 _ _ w472 _]
                seq-local: [_ _ w275 _ _ _ _ _ _] -> [_ _ _ _ w405 _ _ _ _]
                seq-local: [_ _ w268 _ _ _ _ _ _] -> [_ _ _ _ w402 _ _ _ _]
                seq-local: [w250 _ _ _ _ _ _ _ _] -> [_ _ w265 _ _ _ _ _ _]
                seq-local: [w249 _ _ _ _ _ _ _ _] -> [_ _ w264 _ _ _ _ _ _]
                seq-local: [_ _ w263 _ _ _ _ _ _] -> [_ _ _ _ _ _ _ w478 _]
                seq-local: [_ _ _ _ w401 _ _ _ _] -> [_ _ _ _ _ w451 _ w476 _]
                seq-local: [_ _ _ _ w400 _ _ _ _] -> [_ _ _ _ _ _ _ w475 _]
                seq-local: [_ _ _ _ _ _ w458 _ _] -> [_ _ _ _ _ _ _ w466 _]
                seq-local: [_ _ _ w395 _ _ _ _ _] -> [_ _ _ _ _ _ _ _ w618]
                tunnel: w247 -> [_ _ w272 _ w410 _ _ w477 _]
                tunnel: w246 -> [_ _ w273 w398 w409 _ w462 w480 _]
                tunnel: w245 -> [_ _ w274 w397 w408 _ w464 w481 _]
                tunnel: w244 -> [_ _ w271 _ _ _ _ w465 _]
                tunnel: w238 -> [_ _ w270 _ w404 _ _ _ _]
                tunnel: w243 -> [_ _ _ _ w403 _ _ _ _]
                tunnel: w242 -> [_ _ w269 _ _ _ _ _ _]
                tunnel: [_ _ _ _ w400 _ _ _ _] -> w239
                tunnel: [_ _ w263 _ _ _ _ _ _] -> w241
                tunnel: [_ _ _ _ w401 _ _ _ _] -> w240
                tunnel: w238 -> [_ _ _ _ _ _ _ w479 _]
                tunnel: w237 -> [_ _ _ _ _ _ _ w474 _]
                tunnel: w235 -> [_ _ w262 w394 _ _ w463 w473 _]
                tunnel: [_ _ _ _ _ _ _ w471 _] -> w236
                tunnel: [_ _ _ _ _ _ _ w469 _] -> w234
                tunnel: w233 -> [_ _ _ _ w399 _ _ w468 _]
                tunnel: w232 -> [_ _ _ w391 _ _ _ _ w616]
                tunnel: w231 -> [_ _ _ _ _ _ _ w467 _]
                frame #0 {
                  # "generate initial aberration (aberr to correct)"
                  n61 = case shown="\"randomly generated\"" "?" {
                    tunnel: ["Initial Zer index" w256] -> w250
                    tunnel: ["Initial Zer coeff" w255] -> w249
                    tunnel: "max random order" -> [_ w254]
                    frame "input manually " {
                    }
                    frame "randomly generated" {
                      # "generate random zernike index and coefficient arrays"
                      n62 = call "Random Aberration Array Generator.vi"("max random order"=w254, "aberration tolerance"="aberration tolerance", "aberration threshold"="aberration threshold") -> ("Zer coeff"=w255:dbl[], "Zer index (starting from 3)"=w256:dbl[])  [unwired: 7 in]
                      "Initial Zer index (starting from 4)\nrandomly generated" <- w256
                      "Initial Zer coeff\nRandomly generated" <- w255
                    }
                  }
                }
                frame #1 {
                  # "read in offset command"
                  n63 = call-poly <vilib>:"Read From Spreadsheet File.vi"("format (%.3f)"="%.8f", "file path (dialog if empty)"="Offset command file") -> ("first row"=w259:dbl[])  [unwired: 5 in, 4 out]
                }
                frame #2 {
                  w284 = 0.0
                  # "ini zern coeff"
                  # "offset+ini command"
                  # "Zern coeff"
                  # "Zern index"
                  # "calculate the command:\nfor phase diversity"
                  n64 = Array Size(array="Zern index in 2") -> (size(s)=w282:i32)
                  n65 = call-poly <vilib>:"Ramp Pattern.vi"("start"=w284, "end"=w284, "samples"=w282) -> ("Ramp Pattern"=w281:dbl[])  [unwired: 7 in, 1 out]
                  n66 = Build Array(w281, "Zern index in 2", "Zern index in 3", "Zern index in 4", "Zern index in 5") -> (w266:T4)
                  n67 = Build Array(w281, "Zern coef in 2", "Zern coef in 3", "Zern coef in 4", "Zern coef in 5") -> (w285:T4)
                  n68 = Transpose Matrix(1:w285) -> (0:w278:T4)
                  n69 = Transpose Matrix(1:w266) -> (0:w276:T4)
                  n70 = Array Size(array=w266) -> (size(s)=w267:i32[])
                  n71 = Index Array(array=w267, index=1) -> (element=w275:i32)
                  "# of Phase" <- w275
                  n72 = stacked-sequence {
                    seq-local: [w294 _ _] -> [_ w312 w378]
                    seq-local: [w295 _ _] -> [_ w306 _]
                    seq-local: [_ w305 _] -> [_ _ w375]
                    seq-local: [w293 _ _] -> [_ w304 _]
                    tunnel: w275 -> [_ w317 _]
                    tunnel: w265 -> [w302 _ _]
                    tunnel: w264 -> [w301 w307 _]
                    tunnel: w270 -> [w300 w314 _]
                    tunnel: w279 -> [w298 _ _]
                    tunnel: w276 -> [_ w316 _]
                    tunnel: w278 -> [_ w315 _]
                    tunnel: w271 -> [w297 w313 _]
                    tunnel: [_ w311 _] -> w277
                    tunnel: w274 -> [_ w309 w376]
                    tunnel: w273 -> [_ w310 w377]
                    tunnel: w272 -> [_ w308 _]
                    tunnel: w269 -> [w296 _ _]
                    tunnel: [_ _ w374] -> w268
                    tunnel: [w294 _ _] -> w263
                    tunnel: w262 -> [_ w303 w372]
                    frame #0 {
                      n73 = call "zern2command_test.vi"("Initial haso file"=w297, "error in (no error)"=w296, "interaction matrix file"=w300, "Zern coef in"=w301, "Zern index in"=w302) -> ("error out"=w295:errorcluster, "Zern coef out"=w293:sgl[], "Offset positions"=w299:sgl[])  [unwired: 4 in]
                      n74 = Add(x=w299, y=w298) -> (x+y=w294:dbl[])
                    }
                    frame #1 {
                      n75 = for {
                        N: w317 -> [w320]
                        tunnel: w316 -> [w333] mode=indexing
                        tunnel: w315 -> [w332] mode=indexing
                        tunnel: w314 -> [w331]
                        tunnel: w313 -> [w330]
                        tunnel: w312 -> [w329]
                        tunnel: [w328] -> w311 mode=indexing
                        tunnel: w310 -> [w327]
                        tunnel: w309 -> [w326]
                        tunnel: w308 -> [w325]
                        tunnel: w307 -> [w324]
                        tunnel: w306 -> [w323]
                        tunnel: [w322] -> w305
                        tunnel: w304 -> [w319]
                        tunnel: w303 -> [w318]
                        i -> [w321]
                        n76 = stacked-sequence {
                          seq-local: [w339 _] -> [_ w358]
                          seq-local: [w335 _] -> [_ w357]
                          tunnel: w333 -> [w348 _]
                          tunnel: w332 -> [w347 _]
                          tunnel: w331 -> [w346 _]
                          tunnel: w330 -> [w345 _]
                          tunnel: w329 -> [w343 _]
                          tunnel: [w342 _] -> w328
                          tunnel: w327 -> [_ w360]
                          tunnel: w326 -> [_ w359]
                          tunnel: w325 -> [_ _]
                          tunnel: w321 -> [w341 _]
                          tunnel: w324 -> [w337 _]
                          tunnel: w323 -> [w336 _]
                          tunnel: [_ w356] -> w322
                          tunnel: w321 -> [_ _]
                          tunnel: w320 -> [_ _]
                          tunnel: w319 -> [w334 _]
                          tunnel: w318 -> [_ w353]
                          frame #0 {
                            n77 = Equal To 0?(x=w341) -> (x = 0?=w340:bool)
                            n78 = call "zern2command_test.vi"("Initial haso file"=w345, "error in (no error)"=w336, "interaction matrix file"=w346, "Zern coef in"=w347, "Zern index in"=w348) -> ("error out"=w335:errorcluster, "Zern coef out"=w338:sgl[], "Offset positions"=w344:sgl[])  [unwired: 4 in]
                            n79 = case shown="True" w340 {
                              tunnel: [w349 w350] -> w339
                              tunnel: w338 -> [w349 _]
                              tunnel: w337 -> [_ _]
                              tunnel: w334 -> [_ w350]
                              frame False {
                              }
                              frame True {
                              }
                            }
                            n80 = Add(x=w343, y=w344) -> (x+y=w342:dbl[])
                          }
                          frame #1 {
                            n81 = Number To Fractional String(number=w353, precision (6)=0) -> (F-format string=w352:string)  [unwired: 2 in]
                            n82 = Concatenate Strings(w360, w359, "_", w352, "_coeff.txt") -> (w368:string)
                            n83 = String To Path(string=w368) -> (path=w367:path)
                            n84 = Open/Create/Replace File(file path (use dialog)=w367, error in=w357, operation (0:open)=3) -> (refnum out=w364:refnum<file>, error out=w365:errorcluster)  [unwired: 3 in, 1 out]
                            n85 = Array To Spreadsheet String(array=w358, 3:"%f") -> (spreadsheet string=w355:string)  [unwired: 1 in]
                            n86 = Set File Position(refnum=w364, from (0:start)=1, error in=w365) -> (refnum out=w362:refnum<file>, error out=w361:errorcluster)  [unwired: 1 in]
                            n87 = Write to Text File(file (use dialog)=w362, text=w355, error in=w361) -> (error out=w356:errorcluster)  [unwired: 1 in, 2 out]
                          }
                        }
                      }
                    }
                    frame #2 {
                      n88 = Number To Fractional String(number=w372, precision (6)=0) -> (F-format string=w371:string)  [unwired: 2 in]
                      n89 = Concatenate Strings(w377, w376, "_", w371, "_IniAbr+offset.txt") -> (w387:string)
                      n90 = String To Path(string=w387) -> (path=w385:path)
                      n91 = Open/Create/Replace File(file path (use dialog)=w385, error in=w375, operation (0:open)=3) -> (refnum out=w382:refnum<file>, error out=w383:errorcluster)  [unwired: 3 in, 1 out]
                      n92 = Array To Spreadsheet String(array=w378, 3:"%f") -> (spreadsheet string=w389:string)  [unwired: 1 in]
                      n93 = Set File Position(refnum=w382, from (0:start)=1, error in=w383) -> (refnum out=w380:refnum<file>, error out=w379:errorcluster)  [unwired: 1 in]
                      n94 = Write to Text File(file (use dialog)=w380, text=w389, error in=w379) -> (error out=w374:errorcluster)  [unwired: 1 in, 2 out]
                    }
                  }
                }
                frame #3 {
                  # "set andor kinetics and spooling, \nstart acquire and wait for the external trigger"
                  n95 = Number To Fractional String(number=w394, precision (6)=0) -> (F-format string=w392:string)  [unwired: 2 in]
                  n96 = Concatenate Strings(w398, w397, "_PhsDiv_ToBeDeleted_", w392) -> (w395:string)
                  n97 = call "SetSpool_WaitForExtTrigger.vi"("path and name"=w395, "Kinetic Series"=w391) -> ()  [unwired: 10 in]
                }
                frame #4 {
                  # "take phase diversity pictures"
                  n98 = for {
                    N: w405 -> [_]
                    tunnel: w410 -> [w421]
                    tunnel: w409 -> [w420]
                    tunnel: w408 -> [w419]
                    tunnel: w404 -> [w418]
                    tunnel: w407 -> [w417]
                    tunnel: w406 -> [w416] mode=indexing
                    tunnel: w403 -> [w415]
                    tunnel: w402 -> [w414]
                    tunnel: [w413] -> w400
                    tunnel: [w412] -> w401
                    tunnel: w399 -> [w411]
                    n99 = stacked-sequence {
                      seq-local: [w422 _] -> [_ w432]
                      tunnel: w421 -> [_ w429]
                      tunnel: w420 -> [_ _]
                      tunnel: w419 -> [_ _]
                      tunnel: w418 -> [_ _]
                      tunnel: w417 -> [_ _]
                      tunnel: w416 -> [w423 _]
                      tunnel: w415 -> [_ w433]
                      tunnel: w414 -> [w424 _]
                      tunnel: [_ w431] -> w413
                      tunnel: [_ w430] -> w412
                      tunnel: w411 -> [w425 _]
                      frame #0 {
                        # "response time of mirror"
                        n100 = call <userlib>:"LVClass_WavefrontCorrector Move to Absolute Position.vi"("WavefrontCorrector in"=w425, "Absolute Positions"=w423, "error in (no error)"=w424) -> ("error out"=w422:errorcluster)  [unwired: 11 in, 1 out]
                        n101 = Add(x=5, y=10) -> (x+y=w426:i32)
                        n102 = Wait (ms)(milliseconds to wait=w426) -> ()  [unwired: 1 out]
                      }
                      frame #1 {
                        n103 = for {
                          N: w429 -> [_]
                          tunnel: w433 -> [w438]
                          tunnel: w432 -> [w437]
                          tunnel: [w436] -> w431
                          tunnel: [w435] -> w430
                          tunnel: w429 -> [w434]
                          n104 = stacked-sequence {
                            tunnel: w438 -> [w443 _]
                            tunnel: w437 -> [w441 _]
                            tunnel: [w440 _] -> w436
                            tunnel: [w439 _] -> w435
                            tunnel: w434 -> [_ w447]
                            frame #0 {
                              n105 = local read "EMCCD trigger port"() -> (w446:tag)
                              n106 = Add(x=w443, y=0.04) -> (x+y=w442:dbl)
                              n107 = Multiply(x=w442, y=1000.0) -> (x*y=w439:dbl)
                              n108 = call "trig EMCCD.vi"("error in (no error)"=w441, "exp time (ms)"=w439, "lines"=w446) -> ("error out"=w440:errorcluster)
                            }
                            frame #1 {
                              n109 = Not Equal?(x=w447, y=1) -> (x != y?=w449:bool)
                              n110 = case shown="True" w449 {
                                frame False {
                                }
                                frame True {
                                n111 = Wait (ms)(milliseconds to wait=50) -> ()  [unwired: 1 out]
                                }
                              }
                            }
                          }
                        }
                      }
                    }
                  }
                }
                frame #5 {
                  # "send out a trigger to EMCCD to end the aquisition."
                  n112 = local read "EMCCD trigger port"() -> (w452:tag)
                  n113 = call "trig EMCCD.vi"("exp time (ms)"=w451, "lines"=w452) -> ()  [unwired: 1 in, 1 out]
                }
                frame #6 {
                  w456 = 0
                  # "save phase diversity pictures:\npictures per phase*number of phases (Eg: 2*5=10 pictures in this file)"
                  n114 = Number To Fractional String(number=w463, precision (6)=w456) -> (F-format string=w461:string)  [unwired: 2 in]
                  n115 = Concatenate Strings(w464, "_", w461) -> (w458:string)
                  "phase diversity file name" <- w458
                  n116 = Concatenate Strings(w458, ".tif") -> (w459:string)
                  n117 = Concatenate Strings(w462, w459) -> (w454:string)
                  n118 = call <userlib>:"SaveAsTiff.vi"("path"=w454, "palette"="C:\\Program Files\\Andor SOLIS\\GREY.PAL", "position"=w456, "type"=1) -> ()  [unwired: 10 in, 2 out]
                }
                frame #7 {
                  # "run matlab correction?"
                  n119 = case shown="True" w474 {
                    tunnel: w480 -> [_ w497]
                    tunnel: w481 -> [_ w496]
                    tunnel: w479 -> [_ w495]
                    tunnel: w478 -> [_ w494]
                    tunnel: w476 -> [_ w493]
                    tunnel: w477 -> [_ w492]
                    tunnel: w475 -> [_ w491]
                    tunnel: w473 -> [_ w490]
                    tunnel: w472 -> [_ _]
                    tunnel: [0 w489] -> w471
                    tunnel: w470 -> [_ w488]
                    tunnel: [errorcluster {"status"=FALSE, "code"=0, "source"=""} ("Error out 2") w487] -> w469
                    tunnel: w468 -> [_ w486]
                    tunnel: w467 -> [_ w485]
                    tunnel: w466 -> [_ _]
                    tunnel: w465 -> [_ w484]
                    frame False {
                    }
                    frame True {
                      # "matlab reconstructed Zern"
                      n120 = stacked-sequence {
                        seq-local: [w515 _ _ _ _ _ _ _ _ _ _] -> [_ _ _ _ _ _ w570 _ _ _ _]
                        seq-local: [w521 _ _ _ _ _ _ _ _ _ _] -> [_ _ _ _ _ _ w566 _ _ _ _]
                        seq-local: [_ _ _ _ w548 _ _ _ _ _ _] -> [_ _ _ _ _ w555 _ _ _ _ _]
                        seq-local: [_ _ w536 _ _ _ _ _ _ _ _] -> [_ _ _ w543 _ _ _ _ _ _ _]
                        seq-local: [_ _ _ w545 _ _ _ _ _ _ _] -> [_ _ _ _ w549 _ _ _ _ _ _]
                        seq-local: [_ w528 _ _ _ _ _ _ _ _ _] -> [_ _ _ _ _ _ _ _ _ _ w605]
                        seq-local: [_ _ _ _ _ _ w559 _ _ _ _] -> [_ _ _ _ _ _ _ w576 _ _ _]
                        tunnel: w497 -> [w520 w531 _ _ _ _ _ _ _ w594 _]
                        tunnel: w496 -> [w514 w530 _ _ _ _ _ _ _ w593 _]
                        tunnel: w495 -> [_ _ _ _ _ _ w569 _ _ _ _]
                        tunnel: w494 -> [_ _ _ _ w550 _ w568 _ _ _ _]
                        tunnel: w493 -> [_ _ _ w547 _ w557 _ w577 w591 _ _]
                        tunnel: w491 -> [_ _ w537 _ _ _ _ _ _ _ _]
                        tunnel: [_ _ _ w546 _ _ _ _ _ _ _] -> _
                        tunnel: w492 -> [_ _ _ w546 _ _ _ w574 _ _ _]
                        tunnel: w490 -> [w512 w529 _ _ _ _ _ _ _ w595 _]
                        tunnel: [w499 _ _ _ _ _ _ _ _ _ _] -> w489
                        tunnel: w488 -> [_ _ w538 _ _ _ _ _ _ _ _]
                        tunnel: [_ _ _ _ _ _ _ w575 _ _ _] -> w487
                        tunnel: w486 -> [_ _ w539 _ w551 _ w562 _ _ _ _]
                        tunnel: w485 -> [_ w532 _ _ _ _ _ _ _ _ w603]
                        tunnel: w484 -> [_ _ _ _ _ _ w558 _ _ _ _]
                        frame #0 {
                          # "MATLAB does the reconstruction, written by Min Guo"
                          # "other parameters are default in this VI"
                          n121 = Number To Fractional String(number=w512, precision (6)=0) -> (F-format string=w510:string)  [unwired: 2 in]
                          n122 = Concatenate Strings(w514, "_", w510) -> (w498:string)
                          n123 = String To Path(string=w520) -> (path=w522:path)
                          n124 = Concatenate Strings(w520, w498) -> (w519:string)
                          n125 = String To Path(string=w519) -> (path=w518:path)
                          n126 = call "recon_zern_fileIO_MATLAB_v2.vi"("Number of Phase"="Number of Phase", "Number for average"="Number for average", "Crop Size of image"="Crop Size of image", "Background Value"="Background Value", "Zernike Order"="Zernike Order", "Use GPU"="Use GPU", "Iteration Number"="Iteration Number", "File Name"=w498, "Gamma Value"="Gamma Value", "Path In"=w522, "Show Input"="Show Input", "Path Out"=w518, "Show Recon"="Show Recon") -> ("Zern coef out"=w516:sgl[], "RMSE Value"=w499:dbl, "error out"=w521:errorcluster)  [unwired: 3 in, 1 out]
                          n127 = case shown="False" "Keep Reconstructed Defocus component?" {
                            tunnel: w516 -> [w523 w527]
                            tunnel: [w523 w524] -> w515
                            frame False {
                            }
                            frame True {
                              n128 = Replace Array Subset(array=w527, new element=0.0, index=2) -> (w524:sgl[])
                            }
                          }
                        }
                        frame #1 {
                          # "set andor kinetics and spooling, \nstart acquire and wait for the external trigger"
                          n129 = Number To Fractional String(number=w529, precision (6)=0) -> (F-format string=w533:string)  [unwired: 2 in]
                          n130 = Concatenate Strings(w531, w530, "_Corr_ToBeDeleted_", w533) -> (w528:string)
                          n131 = call "SetSpool_WaitForExtTrigger.vi"("path and name"=w528, "Kinetic Series"=w532) -> ()  [unwired: 10 in]
                        }
                        frame #2 {
                          # "groundtruth command"
                          # "response time of mirror"
                          n132 = call <userlib>:"LVClass_WavefrontCorrector Move to Absolute Position.vi"("WavefrontCorrector in"=w539, "Absolute Positions"=w538, "error in (no error)"=w537) -> ("error out"=w536:errorcluster)  [unwired: 11 in, 1 out]
                          n133 = Add(x=5, y=10) -> (x+y=w540:i32)
                          n134 = Wait (ms)(milliseconds to wait=w540) -> ()  [unwired: 1 out]
                        }
                        frame #3 {
                          # "take offset/groundtruth picture, only one"
                          n135 = local read "EMCCD trigger port"() -> (w544:tag)
                          n136 = call "trig EMCCD.vi"("error in (no error)"=w543, "exp time (ms)"=w547, "lines"=w544) -> ("error out"=w545:errorcluster)
                        }
                        frame #4 {
                          # "aberrated picture command"
                          # "response time of mirror"
                          n137 = call <userlib>:"LVClass_WavefrontCorrector Move to Absolute Position.vi"("WavefrontCorrector in"=w551, "Absolute Positions"=w550, "error in (no error)"=w549) -> ("error out"=w548:errorcluster)  [unwired: 11 in, 1 out]
                          n138 = Add(x=5, y=10) -> (x+y=w552:i32)
                          n139 = Wait (ms)(milliseconds to wait=w552) -> ()  [unwired: 1 out]
                        }
                        frame #5 {
                          # "take offset+initial aberr picture, only one"
                          n140 = local read "EMCCD trigger port"() -> (w556:tag)
                          n141 = call "trig EMCCD.vi"("error in (no error)"=w555, "exp time (ms)"=w557, "lines"=w556) -> ()  [unwired: 1 out]
                        }
                        frame #6 {
                          w573 = 1
                          # "correction command"
                          # "response time of mirror"
                          n142 = call-poly <vilib>:"Ramp Pattern.vi"("start"=w573, "end"=32, "delta"=w573) -> ("Ramp Pattern"=w571:dbl[])  [unwired: 6 in, 2 out]
                          n143 = call "zern2command_test.vi"("Initial haso file"=w558, "error in (no error)"=w566, "interaction matrix file"=w569, "Zern coef in"=w570, "Zern index in"=w571) -> ("error out"=w560:errorcluster, "Offset positions"=w567:sgl[])  [unwired: 4 in, 1 out]
                          n144 = Add(x=w568, y=w567) -> (x+y=w561:dbl[])
                          n145 = call <userlib>:"LVClass_WavefrontCorrector Move to Absolute Position.vi"("WavefrontCorrector in"=w562, "Absolute Positions"=w561, "error in (no error)"=w560) -> ("error out"=w559:errorcluster)  [unwired: 11 in, 1 out]
                          n146 = Add(x=5, y=10) -> (x+y=w563:i32)
                          n147 = Wait (ms)(milliseconds to wait=w563) -> ()  [unwired: 1 out]
                        }
                        frame #7 {
                          # "corrected pictures"
                          n148 = for {
                            N: w574 -> [_]
                            tunnel: w577 -> [w581]
                            shift-right: [w579] -> w575
                            shift-left: w576 -> [w580]
                            tunnel: w574 -> [w578]
                            n149 = stacked-sequence {
                              tunnel: w581 -> [w584 _]
                              tunnel: w580 -> [w583 _]
                              tunnel: [w582 _] -> w579
                              tunnel: w578 -> [_ w586]
                              frame #0 {
                                n150 = local read "EMCCD trigger port"() -> (w585:tag)
                                n151 = call "trig EMCCD.vi"("error in (no error)"=w583, "exp time (ms)"=w584, "lines"=w585) -> ("error out"=w582:errorcluster)
                              }
                              frame #1 {
                                n152 = Not Equal?(x=w586, y=1) -> (x != y?=w588:bool)
                                n153 = case shown="True" w588 {
                                frame False {
                                }
                                frame True {
                                n154 = Wait (ms)(milliseconds to wait=50) -> ()  [unwired: 1 out]
                                }
                                }
                              }
                            }
                          }
                        }
                        frame #8 {
                          # "one more trigger to end picture acquisition"
                          n155 = local read "EMCCD trigger port"() -> (w590:tag)
                          n156 = call "trig EMCCD.vi"("exp time (ms)"=w591, "lines"=w590) -> ()  [unwired: 1 in, 1 out]
                        }
                        frame #9 {
                          w598 = 0
                          # "save:\none groundtruth picture\none offset+abrr picture\nPictures per phase*corrected picture"
                          n157 = Number To Fractional String(number=w595, precision (6)=w598) -> (F-format string=w597:string)  [unwired: 2 in]
                          n158 = Concatenate Strings(w593, "_1grdtrth_1abrr_Corr_", w597, ".tif") -> (w602:string)
                          "Corrected Picture name" <- w602
                          n159 = Concatenate Strings(w594, w602) -> (w596:string)
                          n160 = call <userlib>:"SaveAsTiff.vi"("path"=w596, "palette"="C:\\Program Files\\Andor SOLIS\\GREY.PAL", "position"=w598, "type"=1) -> ()  [unwired: 10 in, 2 out]
                        }
                        frame #10 {
                          n161 = case shown="True" TRUE {
                            tunnel: w605 -> [_ w607]
                            tunnel: w603 -> [_ w606]
                            frame False {
                            }
                            frame True {
                              # "delete spooling data"
                              n162 = for {
                                N: w606 -> [_]
                                tunnel: w607 -> [w614]
                                i -> [w612]
                                n163 = Number To Fractional String(number=w612, precision (6)=0) -> (F-format string=w610:string)  [unwired: 2 in]
                                n164 = Concatenate Strings(w614, "000000000", w610, ".dat") -> (w609:string)
                                n165 = String To Path(string=w609) -> (path=w615:path)
                                n166 = Delete(path (use dialog)=w615) -> ()  [unwired: 4 in, 3 out]
                              }
                            }
                          }
                        }
                      }
                    }
                  }
                }
                frame #8 {
                  # "delete spooling data of phase diversity"
                  n167 = case shown="True" TRUE {
                    tunnel: w618 -> [_ w620]
                    tunnel: w616 -> [_ w619]
                    frame False {
                    }
                    frame True {
                      n168 = for {
                        N: w619 -> [_]
                        tunnel: w620 -> [w623]
                        i -> [w622]
                        n169 = Number To Fractional String(number=w622, precision (6)=0) -> (F-format string=w625:string)  [unwired: 2 in]
                        n170 = Concatenate Strings(w623, "000000000", w625, ".dat") -> (w621:string)
                        n171 = String To Path(string=w621) -> (path=w628:path)
                        n172 = Delete(path (use dialog)=w628) -> ()  [unwired: 4 in, 3 out]
                      }
                    }
                  }
                }
              }
            }
          }
          frame #2 {
            # "shut down shutter of 488nm laser"
            n173 = invoke class="MG17Motor" method="SC_Disable"(reference=w632, "lChanID"=w631) -> (reference out=w630:refnum<k7>, "lChanID"=w629:i32)  [unwired: 2 in, 2 out]
          }
          frame #3 {
            # "save the RMS of (calculated zer-real zer)"
            n174 = Concatenate Strings(w635, w634, "_RMSE.txt") -> (w640:string)
            n175 = String To Path(string=w640) -> (path=w639:path)
            n176 = Number To Fractional String(number=w636) -> (F-format string=w637:string[])  [unwired: 3 in]
            n177 = Write to Text File(file (use dialog)=w639, text=w637) -> (error out=w633:errorcluster)  [unwired: 2 in, 2 out]
          }
        }
        n178 = Merge Errors(w189, w188, w183) -> (w182:errorcluster)
        "Error out" <- w182
        n179 = Unbundle(w182) -> ("status"=w178:bool)  [unwired: 2 out]
        n180 = case shown="True" w178 {
          tunnel: [w204 w205] -> w181
          tunnel: w178 -> [w203 w205]
          frame False {
            n181 = Not(x=w203) -> (.not. x?=w204:bool)
          }
          frame True {
          }
        }
        n182 = Or(x=w181, y="?") -> (x .or. y?=w179:bool)
      }
    }
    frame #4 {
      n183 = case shown="True" "Turn off cooler when finished?" {
        frame False {
        }
        frame True {
          n184 = flat-sequence {
            frame #0 {
              n185 = call <userlib>:"CoolerOFF.vi"() -> ()  [unwired: 2 in, 2 out]
            }
            frame #1 {
              # "shut down EMCCD"
              n186 = call <userlib>:"ShutDown.vi"() -> ()  [unwired: 2 in, 2 out]
            }
          }
        }
      }
    }
    frame #5 {
      # "shut down casao"
      n187 = call <userlib>:"LVClass_WavefrontCorrector dtor.vi"("WavefrontCorrector in"=w645, "error in (no error)"=w643) -> ("error out"=w642:errorcluster)  [unwired: 12 in, 1 out]
      n188 = call <userlib>:"LVClass_WavefrontCorrectorSet dtor.vi"("WavefrontCorrectorSet in"=w644, "error in (no error)"=w642) -> ()  [unwired: 12 in, 2 out]
      n189 = invoke class="MG17Motor" method="StopCtrl"(reference=w646) -> ()  [unwired: 2 in, 3 out]
    }
  }
